vi "Running.vi"(0 "DashboardServer in":refnum<class "Dashboard Server.lvclass">, 5 "error in (no error)":errorcluster) -> (14 "DashboardServer out":refnum<class "Dashboard Server.lvclass">, 15 "running":bool, 19 "error out":errorcluster)   [LabVIEW 2016, in "Dashboard Server.lvclass"]
uses:
  Dashboard Server.lvclass
panel:
  out "returnStatus":string
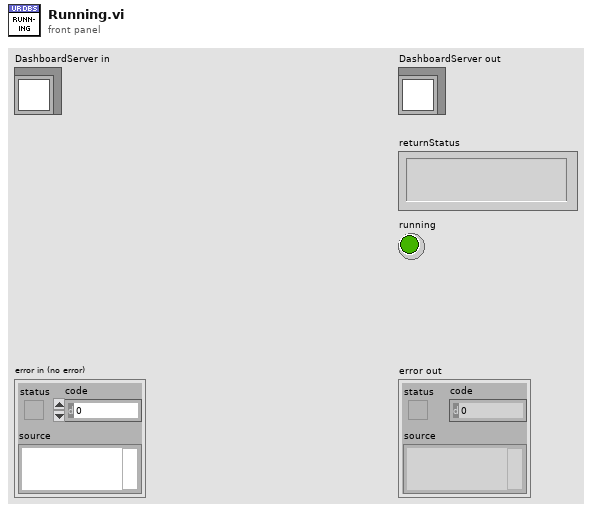
[diagram p1: front panel]
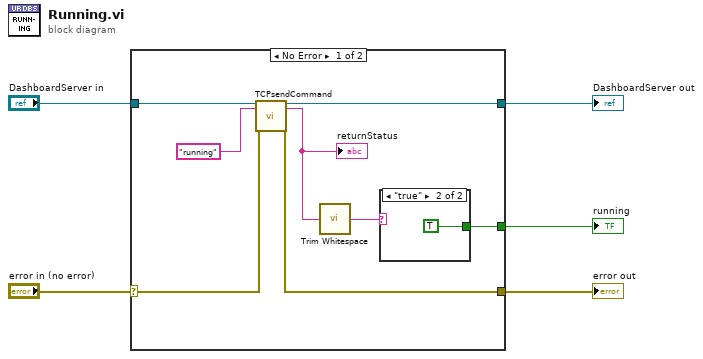
[diagram p0: block diagram]
diagram:
  n1 = case shown="No Error" "error in (no error)" {
    selector: "error in (no error)" -> [w11 w16]
    tunnel: [w10 w16] -> w4
    tunnel: [w12 w15] -> w2
    tunnel: "DashboardServer in" -> [w13 w15]
    tunnel: [w6 _] -> w1
    frame No Error {
      n2 = call-dynamic "TCPsendCommand.vi"("DashboardServer in"=w13, "command"="running", "error in (no error)"=w11) -> ("DashboardServer out"=w12:refnum<class "Dashboard Server.lvclass">, "returnStatus"=w7:string, "error out"=w10:errorcluster)  [unwired: 13 in, 1 out]
      "returnStatus" <- w7
      n3 = call <vilib>:"Trim Whitespace.vi"("string"=w7) -> ("trimmed string"=w8:string)  [unwired: 1 in]
      n4 = case shown="\"true\"" w8 {
        tunnel: [_ TRUE] -> w6
        frame Default {
        }
        frame "true" {
        }
      }
    }
    frame Error {
    }
  }
  "error out" <- w4
  "DashboardServer out" <- w2
  "running" <- w1
